vi "REWORK_display_single_message.vi"(8 "error_in":errorcluster, 11 "message_history_buffer_element":T1) -> (0 "error_out":errorcluster)   [LabVIEW 2019]
uses:
  FGV/DIAGNOSTICS_message_history_buffer/REWORK_DIAGNOSTICS_message_history_buffer_all_info.ctl
  _misc/DIAGNOSTICS_message_type.ctl
  FGV_REWORK_DIAGNOSTICS_single_message_display.ctl
  _misc/AULocalize/SubVIs/RegisterVI.vi
panel:
  in  "single_message_display":i32(listbox)
  in  "STOP":bool
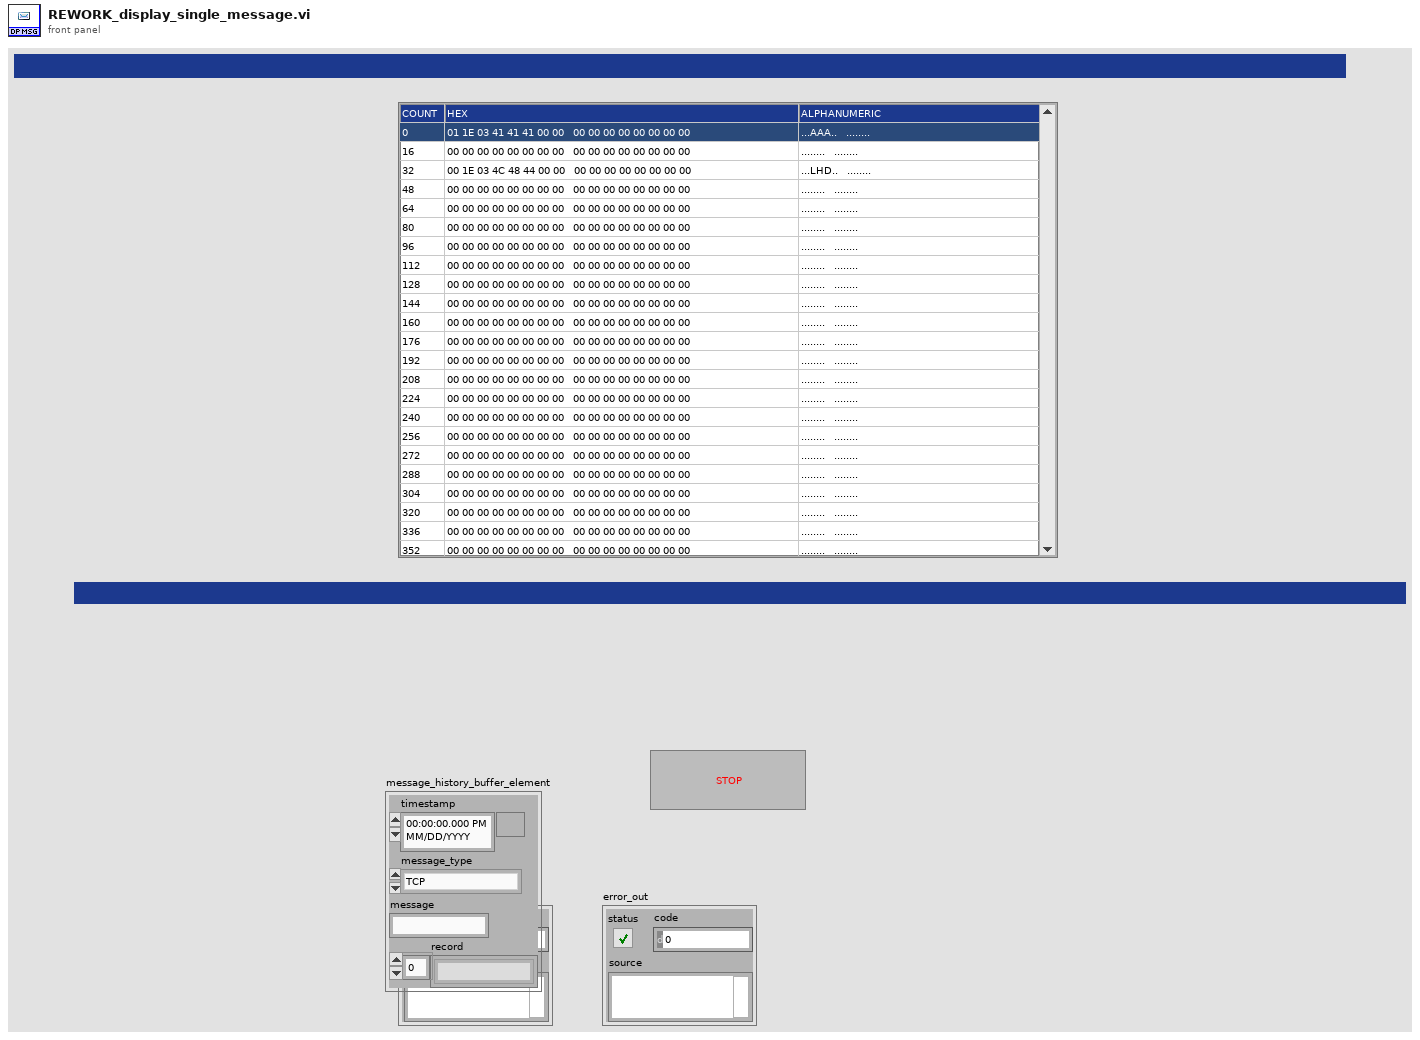
[diagram p1: front panel]
types:
  T1 = typedef "REWORK_DIAGNOSTICS_message_history_buffer_all_info.ctl" = cluster{"timestamp":timestamp, "message_type":T2, "message":string, "record":string[]}
  T2 = typedef "DIAGNOSTICS_message_type.ctl" = enum16{"TCP", "SQL"}
  T3 = typedef "FGV_REWORK_DIAGNOSTICS_single_message_display.ctl" = enum16{"initialize", "display_message"}
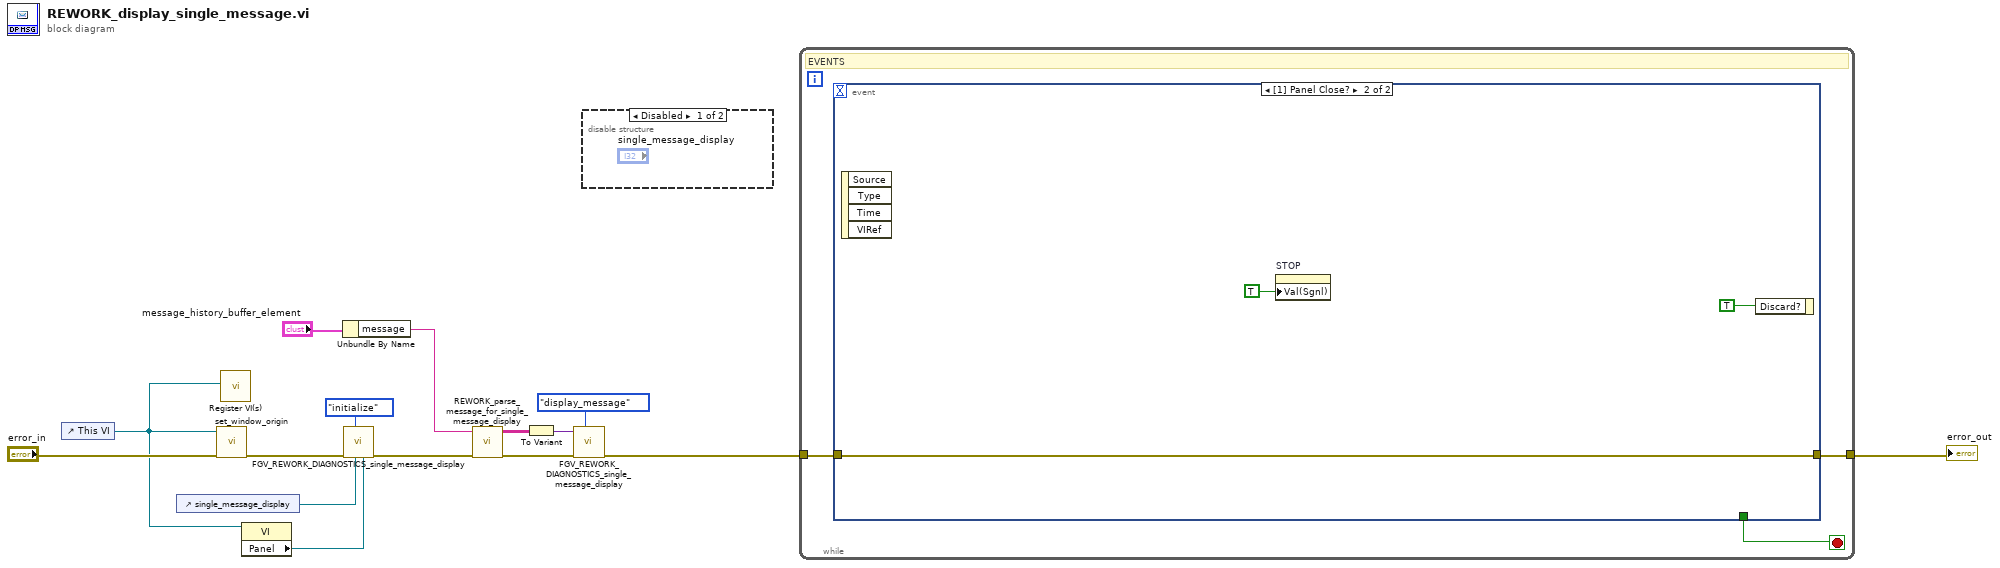
[diagram p0: block diagram]
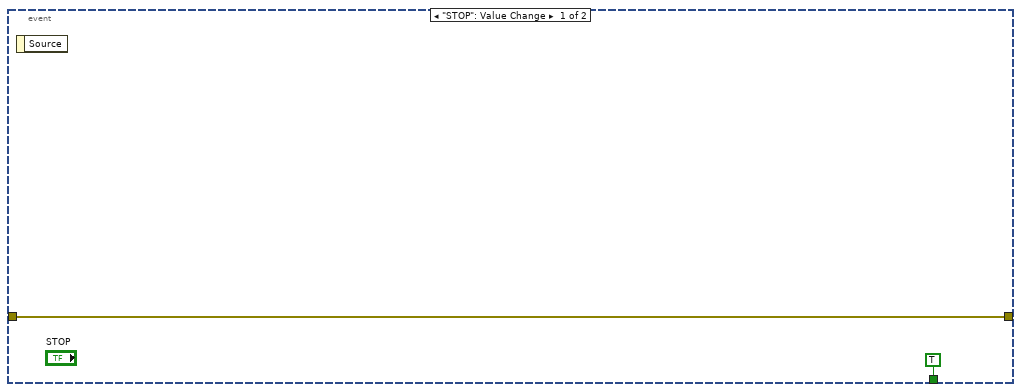
[diagram p3: hidden frame]
diagram:
  n1 = control-ref of="This VI"() -> (w1:refnum<vi>)
  n2 = control-ref of="single_message_display"() -> (w10:refnum<vi>)
  n3 = call "set_window_origin.vi"("error_in"="error_in", "this_vi_reference"=w1) -> ("error_out"=w11:errorcluster)  [unwired: 9 in]
  n4 = call-poly "Register VI(s).vi"("VI Ref"=w1) -> ()  [unwired: 9 in, 2 out]
  n5 = property class="VI"(reference=w1) -> ("Panel"=w9:refnum<vi>)  [unwired: 1 in, 2 out]
  n6 = Unbundle By Name("message_history_buffer_element") -> ("message"=w12:string)
  n7 = call "FGV_REWORK_DIAGNOSTICS_single_message_display.vi"("front_panel_reference"=w9, "SQL_listbox_reference"=w10, "options"=FGV_REWORK_DIAGNOSTICS_single_message_display."initialize", "error_in"=w11) -> ("error_out"=w6:errorcluster)  [unwired: 7 in]
  n8 = call "REWORK_parse_message_for_single_message_display.vi"("error_in"=w6, "message"=w12) -> ("error_out"=w5:errorcluster, "parsed_message"=w3:string[][])  [unwired: 8 in]
  n9 = To Variant(anything=w3) -> (Variant=w4:variant)
  n10 = call "FGV_REWORK_DIAGNOSTICS_single_message_display.vi"("options"=FGV_REWORK_DIAGNOSTICS_single_message_display."display_message", "error_in"=w5, "input"=w4) -> ("error_out"=w2:errorcluster)  [unwired: 8 in]
  n11 = disable-structure shown="Disabled" {
    frame Disabled {
    }
    frame Enabled {
    }
  }
  n12 = while {
    tunnel: [w18] -> w15
    tunnel: w2 -> [w16]
    stop <- w17 stop-if-true
    # "EVENTS"
    n13 = event shown="[1] Panel Close?" {
      selector: _ -> [_ _]
      dyn-events: _ -> [_ _]
      timeout: _ -> [_ _]
      tunnel: [TRUE _] -> w17
      tunnel: w16 -> [w20 w23]
      tunnel: [w20 w23] -> w18
      event "STOP": Value Change {
        n14 = event-data() -> ()  [unwired: 1 in, 1 out]
      }
      event Panel Close? {
        n15 = event-data() -> ()  [unwired: 1 in, 4 out]
        n16 = property on="STOP" class="Bool (strict)"("Val(Sgnl)"=TRUE ("Value (Signaling)")) -> ()  [unwired: 2 in, 2 out]
        n17 = event-data("Discard?"=TRUE) -> ()  [unwired: 1 in, 1 out]
      }
    }
  }
  "error_out" <- w15
